vi "PicoScope3000aWrap.vi"(4 "Enabled Array":i16[](array[numeric]), 5 "Device Info":T1, 6 "handle in":i16, 7 "error in (no error)":errorcluster) -> (0 "deviceIndex":u16, 2 "handle out":i16, 3 "error out":errorcluster)   [LabVIEW 2010]
uses:
  ps3000aWrap.dll
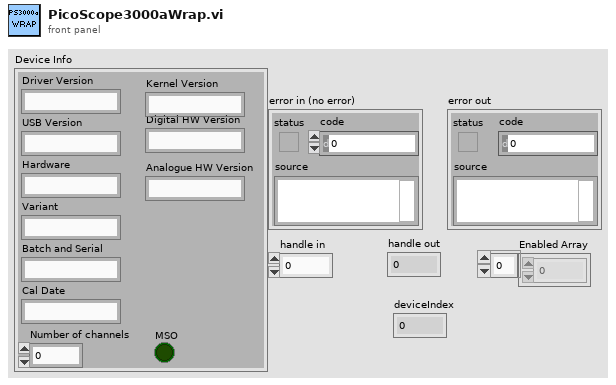
[diagram p1: front panel]
types:
  T1 = cluster{"Driver Version":string, "USB Version":string, "Hardware":string, "Variant":string, "Batch and Serial":string, "Cal Date":string, "Kernel Version":string, "Digital HW Version":string, "Analogue HW Version":string, "MSO":bool, "Number of channels":i16}
  T2 = cluster{"status":bool, "code":u32, "source":string}
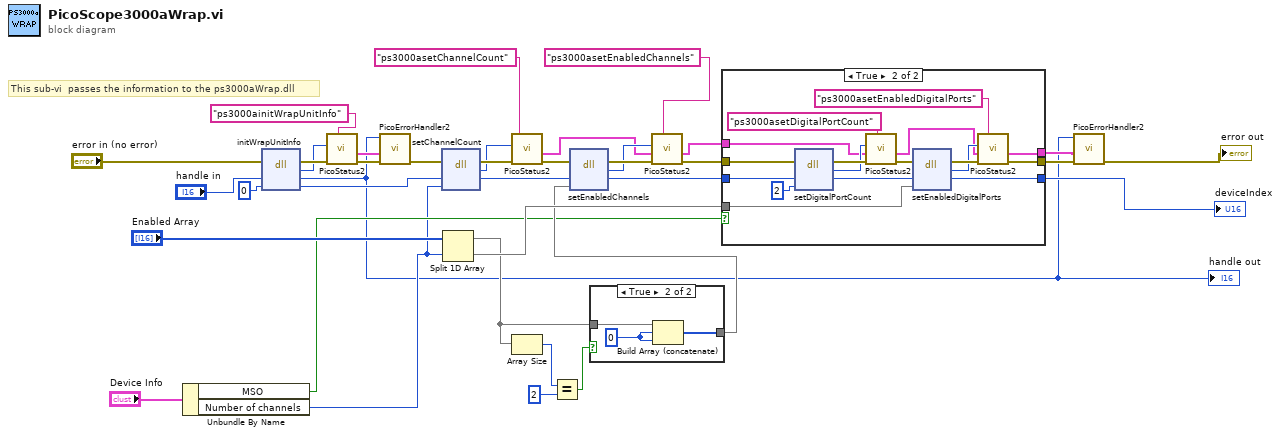
[diagram p0: block diagram]
diagram:
  # "This sub-vi  passes the information to the ps3000aWrap.dll"
  n1 = Unbundle By Name("Device Info") -> ("MSO"=w11:bool, "Number of channels"=w10:i16)
  n2 = dll-call lib="ps3000aWrap.dll" fn="initWrapUnitInfo"(error in="error in (no error)", "handle"="handle in", "deviceIndex"=u16 0) -> (error out=w30:errorcluster, "Pico Status"=w29:u32, "handle"=w2:i16, "deviceIndex"=w34:u16)  [unwired: 2 in, 1 out]
  "handle out" <- w2
  n3 = call "PicoStatus2.vi"("PICO source"="ps3000ainitWrapUnitInfo" ("source"), "Error in"=w30, "PICO STATUS"=w29) -> ("error out"=w4:errorcluster, "PICO_STATUS out"=w3:T2)  [unwired: 5 in]
  n4 = call "PicoErrorHandler2.vi"("error in (no error)"=w4, "PICO_STATUS in"=w3, "handle In"=w2) -> ("error out"=w1:errorcluster)  [unwired: 8 in]
  n5 = dll-call lib="ps3000aWrap.dll" fn="setChannelCount"(error in=w1, "deviceIndex"=w34, "channel count"=w10) -> (error out=w27:errorcluster, "Pico Status"=w26:u32, "deviceIndex"=w37:u16)  [unwired: 3 in, 1 out]
  n6 = Split 1D Array(array="Enabled Array", index=w10) -> (first subarray=w8:i16[], second subarray=w17:i16[])
  n7 = call "PicoStatus2.vi"("PICO source"="ps3000asetChannelCount" ("source"), "Error in"=w27, "PICO STATUS"=w26) -> ("error out"=w28:errorcluster, "PICO_STATUS out"=w5:T2)  [unwired: 5 in]
  n8 = Array Size(array=w8) -> (size(s)=w9:i32)
  n9 = Equal?(x=w9, y=2) -> (x = y?=w15:bool)
  n10 = case shown="True" w15 {
    tunnel: w8 -> [w38 w41]
    tunnel: [w38 w39] -> w13
    frame False {
    }
    frame True {
      w40 = i16 0 ("y")
      n11 = Build Array (concatenate)(w41, w40, w40) -> (w39:i16[])
    }
  }
  n12 = dll-call lib="ps3000aWrap.dll" fn="setEnabledChannels"(error in=w28, "deviceIndex"=w37, "EnabledChannels"=w13) -> (error out=w25:errorcluster, "Pico Status"=w23:u32, "deviceIndex"=w33:u16)  [unwired: 3 in, 1 out]
  n13 = call "PicoStatus2.vi"("PICO source"="ps3000asetEnabledChannels" ("source"), "Error in"=w25, "PICO_STATUS in"=w5, "PICO STATUS"=w23) -> ("error out"=w24:errorcluster, "PICO_STATUS out"=w6:T2)  [unwired: 4 in]
  n14 = case shown="True" w11 {
    tunnel: w24 -> [w44 w61]
    tunnel: [w44 w53] -> w18
    tunnel: w33 -> [w43 w60]
    tunnel: [w43 w57] -> w32
    tunnel: w17 -> [_ w48]
    tunnel: [w42 w47] -> w7
    tunnel: w6 -> [w42 w45]
    frame False {
    }
    frame True {
      n15 = dll-call lib="ps3000aWrap.dll" fn="setDigitalPortCount"(error in=w61, "deviceIndex"=w60, "DigitalPortCount"=i16 2) -> (error out=w56:errorcluster, "Pico Status"=w55:u32, "deviceIndex"=w58:u16)  [unwired: 3 in, 1 out]
      n16 = call "PicoStatus2.vi"("PICO source"="ps3000asetDigitalPortCount" ("source"), "Error in"=w56, "PICO_STATUS in"=w45, "PICO STATUS"=w55) -> ("error out"=w51:errorcluster, "PICO_STATUS out"=w46:T2)  [unwired: 4 in]
      n17 = dll-call lib="ps3000aWrap.dll" fn="setEnabledDigitalPorts"(error in=w51, "deviceIndex"=w58, "EnabledDigitalChannels"=w48) -> (error out=w54:errorcluster, "Pico Status"=w52:u32, "deviceIndex"=w57:u16)  [unwired: 3 in, 1 out]
      n18 = call "PicoStatus2.vi"("PICO source"="ps3000asetEnabledDigitalPorts" ("source"), "Error in"=w54, "PICO_STATUS in"=w46, "PICO STATUS"=w52) -> ("error out"=w53:errorcluster, "PICO_STATUS out"=w47:T2)  [unwired: 4 in]
    }
  }
  "deviceIndex" <- w32
  n19 = call "PicoErrorHandler2.vi"("error in (no error)"=w18, "PICO_STATUS in"=w7, "handle In"=w2) -> ("error out"=→"error out":errorcluster)  [unwired: 8 in]
